vi "Configuration Version to Configuration Info Typedef.vi"(11 "configuration version":cluster{"major":u32, "minor":u32, "fix":u32}) -> (3 "version info":T1)   [LabVIEW 2020, in "DSF Shared.lvlib"]
uses:
  DSF Shared.lvlib
  Includes/DSF Core.lvlibp/Typedefs/DSF Version Info.ctl
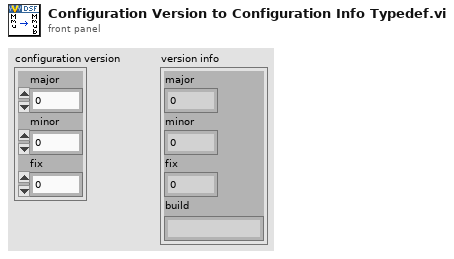
[diagram p1: front panel]
types:
  T1 = typedef "DSF Core.lvlibp/DSF Version Info.ctl" = cluster{"major":u32, "minor":u32, "fix":u32, "build":string}
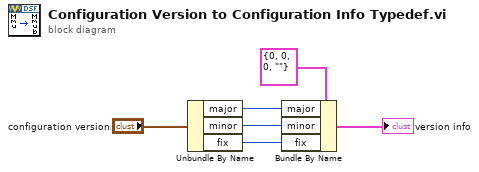
[diagram p0: block diagram]
diagram:
  n1 = Unbundle By Name("configuration version") -> ("major"=w3:u32, "minor"=w4:u32, "fix"=w5:u32)
  n2 = Bundle By Name(cluster=T1 {"major"=0, "minor"=0, "fix"=0, "build"=""} ("version"), "major"=w3, "minor"=w4, "fix"=w5) -> (→"version info":T1)
